vi "Test-1.vi"() -> ()   [LabVIEW 2011]
uses:
  VIs/_USB_CAN_T_R_Unit_.ctl
panel:
  in  "数组":T1[](array[typedef])
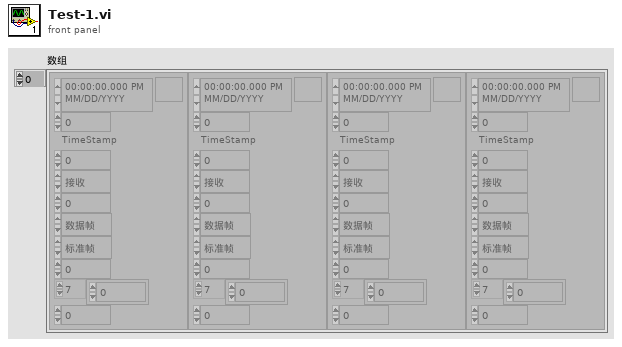
[diagram p1: front panel]
types:
  T1 = typedef "_USB_CAN_T_R_Unit_.ctl" = cluster{"time":timestamp, "channel":u16, "TimeStamp":u32, "tr":enum16{"接收", "发送"}, "id":u32, "Type":enum16{"数据帧", "远程帧"}, "Format":enum16{"标准帧", "扩展帧"}, "len":u8, "data":u8[], "sysTime":u32}
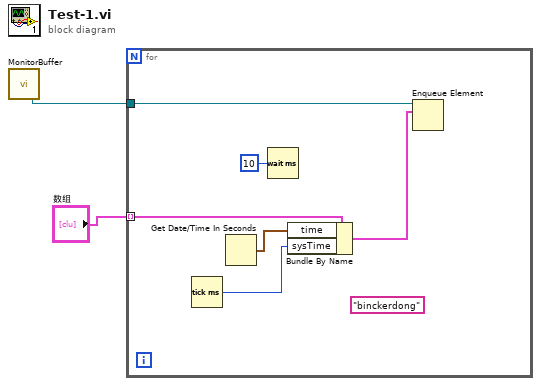
[diagram p0: block diagram]
diagram:
  n1 = call "MonitorBuffer.vi"() -> ("USB_CAN_M_BUF"=w2:refnum<queue>)  [unwired: 1 in]
  n2 = for {
    tunnel: w2 -> [w8]
    tunnel: "数组" -> [w4] mode=indexing
    (unwired) "binckerdong"
    n3 = Tick Count (ms)() -> (millisecond timer value=w5:u32)
    n4 = Get Date/Time In Seconds() -> (seconds since 1Jan1904=w7:timestamp)
    n5 = Wait (ms)(milliseconds to wait=u32 10 ("等待时间（毫秒）")) -> ()  [unwired: 1 out]
    n6 = Bundle By Name(cluster=w4, "time"=w7, "sysTime"=w5) -> (w6:T1)
    n7 = Enqueue Element(queue=w8, element=w6) -> ()  [unwired: 2 in, 3 out]
  }
